vi "calculos_acel_desl_velo.vi"(8 "Clean Graph":bool, 9 "Joint Number":dbl, 10 "TimeStamp":dbl, 11 "Joints":dbl[](array[numeric])) -> (1 "Aceleração":dbl[](array[numeric]), 2 "Velocidade":dbl[](array[numeric]), 3 "Deslocamento":dbl[](array[numeric]))   [LabVIEW 2016]
uses:
  Software_TCC/historico_dados.vi
panel:
  out "Aceleração":dbl[](array[numeric])
  out "Velocidade":dbl[](array[numeric])
  out "Deslocamento":dbl[](array[numeric])
  out "size(s)":i32[](array[numeric])
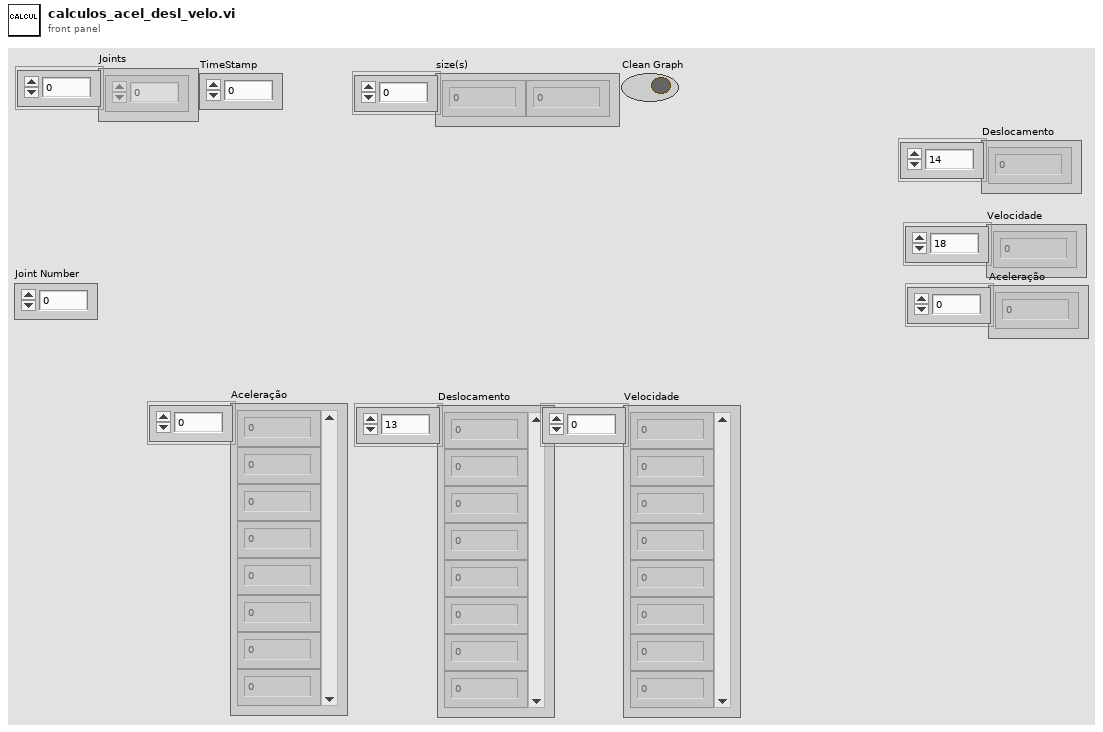
[diagram p1: front panel]
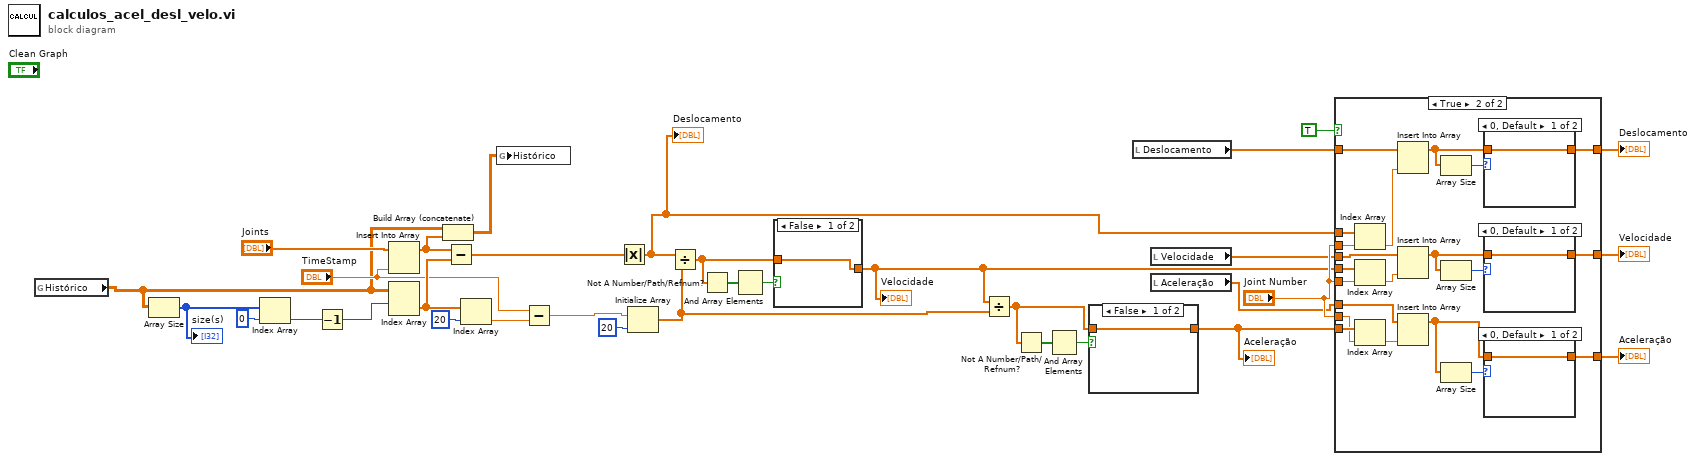
[diagram p0: block diagram]
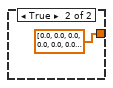
[diagram p2: hidden frame]
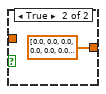
[diagram p3: hidden frame]
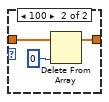
[diagram p5: hidden frame]
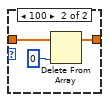
[diagram p6: hidden frame]
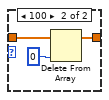
[diagram p7: hidden frame]
diagram:
  n1 = global read "historico_dados.vi" "Histórico"() -> (w2:dbl[][])
  n2 = Array Size(array=w2) -> (size(s)=w33:i32[])
  "size(s)" <- w33
  n3 = Index Array(array=w33, index=0) -> (element=w15:i32)
  n4 = Decrement(x=w15) -> (x-1=w14:i32)
  n5 = Insert Into Array(array="Joints", new element="TimeStamp") -> (w19:dbl[])  [unwired: 1 in]
  n6 = Index Array(array=w2, index (row)=w14) -> (element=w31:dbl[])  [unwired: 1 in]
  n7 = Build Array (concatenate)(w2, w19) -> (w1:dbl[][])
  n8 = Subtract(x=w19, y=w31) -> (x-y=w18:dbl[])
  n9 = Index Array(array=w31, index=20) -> (element=w29:dbl)
  n10 = global write "historico_dados.vi" "Histórico"(w1) -> ()
  n11 = Subtract(x="TimeStamp", y=w29) -> (x-y=w6:dbl)
  n12 = Absolute Value(x=w18) -> (abs(x)=w5:dbl[])
  "Deslocamento" <- w5
  n13 = Initialize Array(w6, 20 ("dimension size")) -> (w3:dbl[])
  n14 = Divide(x=w5, y=w3) -> (x/y=w11:dbl[])
  n15 = Not A Number/Path/Refnum?(number/path/refnum=w11) -> (NaN/Path/Refnum?=w13:bool[])
  n16 = And Array Elements(Boolean array=w13) -> (logical AND=w12:bool)
  n17 = case shown="False" w12 {
    tunnel: [w34 dbl[] [0.0, 0.0, 0.0, 0.0, 0.0, 0.0, 0.0, 0.0, 0.0, 0.0, 0.0, 0.0, 0.0, 0.0, 0.0, 0.0, 0.0, 0.0, 0.0, 0.0, 0.0]] -> w4
    tunnel: w11 -> [w34 _]
    frame False {
    }
    frame True {
    }
  }
  "Velocidade" <- w4
  n18 = Divide(x=w4, y=w3) -> (x/y=w9:dbl[])
  n19 = Not A Number/Path/Refnum?(number/path/refnum=w9) -> (NaN/Path/Refnum?=w10:bool[])
  n20 = And Array Elements(Boolean array=w10) -> (logical AND=w7:bool)
  n21 = case shown="False" w7 {
    tunnel: [w36 dbl[] [0.0, 0.0, 0.0, 0.0, 0.0, 0.0, 0.0, 0.0, 0.0, 0.0, 0.0, 0.0, 0.0, 0.0, 0.0, 0.0, 0.0, 0.0, 0.0, 0.0, 0.0]] -> w8
    tunnel: w9 -> [w36 _]
    frame False {
    }
    frame True {
    }
  }
  "Aceleração" <- w8
  n22 = local read "Deslocamento"() -> (w22:dbl[])
  n23 = local read "Velocidade"() -> (w21:dbl[])
  n24 = local read "Aceleração"() -> (w20:dbl[])
  n25 = case shown="True" TRUE {
    tunnel: w5 -> [_ w61]
    tunnel: w4 -> [_ w60]
    tunnel: w8 -> [_ w59]
    tunnel: "Joint Number" -> [_ w58]
    tunnel: "Joint Number" -> [_ w57]
    tunnel: "Joint Number" -> [_ w56]
    tunnel: w22 -> [w40 w55]
    tunnel: w21 -> [w39 w52]
    tunnel: w20 -> [w38 w49]
    tunnel: [w40 w53] -> w25
    tunnel: [w39 w50] -> w24
    tunnel: [w38 w47] -> w23
    frame False {
    }
    frame True {
      n26 = Index Array(array=w61, index=w56) -> (element=w54:dbl)
      n27 = Index Array(array=w60, index=w57) -> (element=w51:dbl)
      n28 = Index Array(array=w59, index=w58) -> (element=w48:dbl)
      n29 = Insert Into Array(array=w55, new element=w54) -> (w46:dbl[])  [unwired: 1 in]
      n30 = Insert Into Array(array=w52, new element=w51) -> (w45:dbl[])  [unwired: 1 in]
      n31 = Insert Into Array(array=w49, new element=w48) -> (w44:dbl[])  [unwired: 1 in]
      n32 = Array Size(array=w46) -> (size(s)=w43:i32)
      n33 = Array Size(array=w45) -> (size(s)=w41:i32)
      n34 = Array Size(array=w44) -> (size(s)=w42:i32)
      n35 = case shown="0, Default" w43 {
        tunnel: [w62 w64] -> w53
        tunnel: w46 -> [w62 w63]
        frame 0, Default {
        }
        frame 100 {
          n36 = Delete From Array(array=w63, index=0) -> (array with subset deleted=w64:dbl[])  [unwired: 1 in, 1 out]
        }
      }
      n37 = case shown="0, Default" w41 {
        tunnel: [w66 w69] -> w50
        tunnel: w45 -> [w66 w67]
        frame 0, Default {
        }
        frame 100 {
          n38 = Delete From Array(array=w67, index=0) -> (array with subset deleted=w69:dbl[])  [unwired: 1 in, 1 out]
        }
      }
      n39 = case shown="0, Default" w42 {
        tunnel: [w70 w72] -> w47
        tunnel: w44 -> [w70 w71]
        frame 0, Default {
        }
        frame 100 {
          n40 = Delete From Array(array=w71, index=0) -> (array with subset deleted=w72:dbl[])  [unwired: 1 in, 1 out]
        }
      }
    }
  }
  "Deslocamento" <- w25
  "Velocidade" <- w24
  "Aceleração" <- w23
